vi "TestPlay_Init.vi"(0 "object in":refnum<class "TestPlay.lvclass">, 5 "error in (no error)":errorcluster) -> (14 "object out":refnum<class "TestPlay.lvclass">, 19 "error out":errorcluster)   [LabVIEW 2023, in "TestPlay.lvclass"]
uses:
  TestPlay.lvclass
  Play_class/Play.lvclass
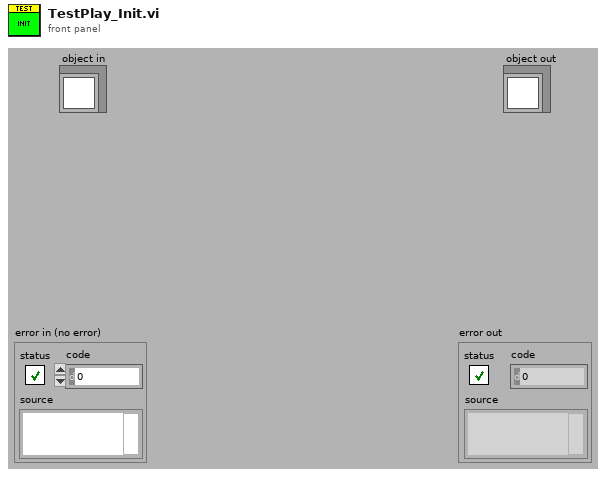
[diagram p1: front panel]
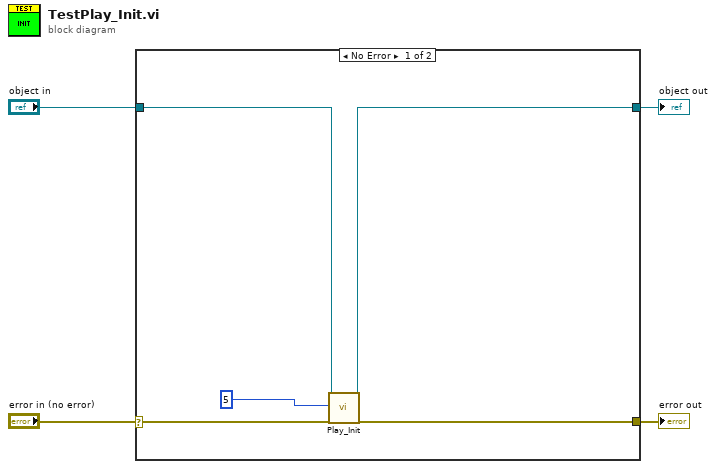
[diagram p0: block diagram]
diagram:
  n1 = case shown="No Error" "error in (no error)" {
    selector: "error in (no error)" -> [w9 w10]
    tunnel: [w5 w11] -> w4
    tunnel: "object in" -> [w7 w11]
    tunnel: [w8 w10] -> w1
    frame No Error {
      n2 = call "Play_Init.vi"("object in"=w7, "number_of_robots"=5, "error in (no error)"=w9) -> ("object out"=w5:refnum<class "TestPlay.lvclass">, "error out"=w8:errorcluster)  [unwired: 15 in]
    }
    frame Error {
    }
  }
  "object out" <- w4
  "error out" <- w1
